vi "checkIfIsFromDirect.vi"(8 "error in (no error)":errorcluster, 10 "Game":refnum<class "Game.lvclass">, 11 "KickToBestRobotTactic in":refnum<class "KickToBestRobotTactic.lvclass">) -> (0 "error out":errorcluster, 2 "FromPreparePass":bool, 3 "KickToBestRobotTactic out":refnum<class "KickToBestRobotTactic.lvclass">)   [LabVIEW 2024, in "KickToBestRobotTactic.lvclass"]
uses:
  KickToBestRobotTactic.lvclass
  Game_class/Game.lvclass
  Game_class/Game.lvclass/Game.ctl
  Team_class/Team.lvclass/Team.ctl
  Playbook_class/Playbook.lvclass/Playbook.ctl
  5RobotsNormalGamePlay_class/5RobotsNormalGamePlay.lvclass/5RobotsNormalGamePlay.ctl
  5RobotsPassGamePlay_class/5RobotsPassGamePlay.lvclass/5RobotsPassGamePlay.ctl
  Playbook_class/Read offensive_plays.vi
  5RobotsNormalGamePlay_class/Read FromPreparePass.vi
  5RobotsPassGamePlay_class/Read FromPreparePass.vi
  Game_class/Read OffensiveTeam.vi
  Team_class/Read OffensivePlay.vi
  Ally_class/Ally.lvclass
  C:/Users/moise/Documents/GitHub/SSL_AI/Team_class/Team.lvclass
  Playbook_class/Playbook.lvclass
  Play_class/Play.lvclass
  TestPlay_class/TestPlay.lvclass
  EnemyPossessionAtEnemyFieldPlay_class/EnemyPossessionAtEnemyFieldPlay.lvclass
  EnemyPossessionAtOurFieldPlay_class/EnemyPossessionAtOurFieldPlay.lvclass
  NormalGamePlay_class/NormalGamePlay.lvclass
  IndirectEnemyPlay_class/IndirectEnemyPlay.lvclass
  PrepareKickoffAllyPlay_class/PrepareKickoffAllyPlay.lvclass
  PrepareKickoffEnemyPlay_class/PrepareKickoffEnemyPlay.lvclass
  KickPenaltyAllyPlay_class/KickPenaltyAllyPlay.lvclass
  PreparePenaltyAllyPlay_class/PreparePenaltyAllyPlay.lvclass
  DirectEnemyPlay_class/DirectEnemyPlay.lvclass
  PreparePenaltyEnemyPlay_class/PreparePenaltyEnemyPlay.lvclass
  BallOutOfFieldPlay_class/BallOutOfFieldPlay.lvclass
  StopOffensivePlay_class/StopOffensivePlay.lvclass
  PassPlay_class/PassPlay.lvclass
  DirectKickPlay_class/DirectKickPlay.lvclass
  HaltPlay_class/HaltPlay.lvclass
  PreparePassPlay_class/PreparePassPlay.lvclass
  PassToStriker_class/PassToStriker.lvclass
  PassTo2ndStriker_class/PassTo2ndStriker.lvclass
  SimplePass_class/SimplePass.lvclass
  PrepareRollToPassPlay_class/PrepareRollToPassPlay.lvclass
  PrepareDoublePassPlay_class/PrepareDoublePassPlay.lvclass
  TableWith2ndStrikerPlay_class/TableWith2ndStrikerPlay.lvclass
  TableWithStrikerPlay_class/TableWithStrikerPlay.lvclass
  PrepareTriplePassPlay_class/PrepareTriplePassPlay.lvclass
  ABCPassPlay_class/ABCPassPlay.lvclass
  PreparePassInGame1_class/PreparePassInGame1.lvclass
  ACBPassPlay_class/ACBPassPlay.lvclass
  PrepareKeeperPassPlay_class/PrepareKeeperPassPlay.lvclass
  KeeperPassToStrikerPlay_class/KeeperPassToStrikerPlay.lvclass
  5RobotsNormalGamePlay_class/5RobotsNormalGamePlay.lvclass
  5RobotsPassGamePlay_class/5RobotsPassGamePlay.lvclass
  5RobotsKeeperGame_class/5RobotsKeeperGame.lvclass
  5PreparePassGamePlay_class/5PreparePassGamePlay.lvclass
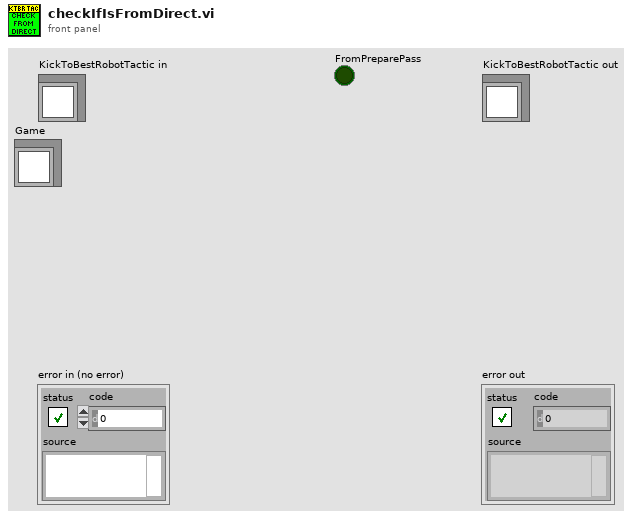
[diagram p1: front panel]
types:
  T1 = typedef "OffensivePlay.ctl" = enum16{"5RobotsPassGamePlay", "5PreparePassGame", "5RobotsKeeperGame", "KeeperPassToStriker", "5RobotsNormalGamePlay", "PrepareKeeperPass", "ACBPass", "ABCPass", "PrepareTriplePass", "TableWithStriker", "TableWith2ndStrikerPlay", "PrepareDoublePass", "PrepareRollToPass", "SimplePass", "PreparePass", "PassToStriker", "BallOutOfField", "PassTo2ndStriker", "StopOffensive", "Prepare Penalty Enemy", "EnemyPossessionAtEnemyField", "EnemyPossesionAtOurField", "TestPlay", "PreparePenaltyAlly", "KickPenaltyAlly", "PrepareKickoffAlly", "PrepareKickoffEnemy", "IndirectEnemy", "DirectEnemy", "PreparePassInGame1", "NormalGame", "DirectKick", "Pass", "Halt", "Timeout", "PassPlay", "PenaltyEnemy"}
  T2 = typedef "offensive_plays.ctl" = cluster{"Play":refnum<class "Play.lvclass">, "TestPlay":refnum<class "TestPlay.lvclass">, "EnemyPossessionAtEnemyFieldPlay":refnum<class "EnemyPossessionAtEnemyFieldPlay.lvclass">, "EnemyPossessionAtOurFieldPlay":refnum<class "EnemyPossessionAtOurFieldPlay.lvclass">, "NormalGamePlay":refnum<class "NormalGamePlay.lvclass">, "IndirectEnemyPlay":refnum<class "IndirectEnemyPlay.lvclass">, "PrepareKickoffAllyPlay":refnum<class "PrepareKickoffAllyPlay.lvclass">, "PrepareKickoffEnemyPlay":refnum<class "PrepareKickoffEnemyPlay.lvclass">, "KickPenaltyAllyPlay":refnum<class "KickPenaltyAllyPlay.lvclass">, "PreparePenaltyAllyPlay":refnum<class "PreparePenaltyAllyPlay.lvclass">, "DirectEnemyPlay":refnum<class "DirectEnemyPlay.lvclass">, "PreparePenaltyEnemyPlay":refnum<class "PreparePenaltyEnemyPlay.lvclass">, "BallOutOfFieldPlay":refnum<class "BallOutOfFieldPlay.lvclass">, "StopOffensivePlay":refnum<class "StopOffensivePlay.lvclass">, "PassPlay":refnum<class "PassPlay.lvclass">, "DirectKickPlay":refnum<class "DirectKickPlay.lvclass">, "HaltPlay":refnum<class "HaltPlay.lvclass">, "PreparePassPlay":refnum<class "PreparePassPlay.lvclass">, "PassToStrikerPlay":refnum<class "PassToStriker.lvclass">, "PassTo2ndStrikerPlay":refnum<class "PassTo2ndStriker.lvclass">, "SimplePassPlay":refnum<class "SimplePass.lvclass">, "PrepareRollToPassPlay":refnum<class "PrepareRollToPassPlay.lvclass">, "PrepareDoublePassPlay":refnum<class "PrepareDoublePassPlay.lvclass">, "TableWith2ndStrikerPlay":refnum<class "TableWith2ndStrikerPlay.lvclass">, "TableWithStrikerPlay":refnum<class "TableWithStrikerPlay.lvclass">, "PrepareTriplePassPlay":refnum<class "PrepareTriplePassPlay.lvclass">, "ABCPassPlay":refnum<class "ABCPassPlay.lvclass">, "PreparePassInGame1":refnum<class "PreparePassInGame1.lvclass">, "ACBPassPlay":refnum<class "ACBPassPlay.lvclass">, "PrepareKeeperPassPlay":refnum<class "PrepareKeeperPassPlay.lvclass">, "KeeperPassToStrikerPlay":refnum<class "KeeperPassToStrikerPlay.lvclass">, "SimplePass":refnum<class "SimplePass.lvclass">, "SimplePass 2":refnum<class "SimplePass.lvclass">, "5RobotsNormalGamePlay":refnum<class "5RobotsNormalGamePlay.lvclass">, "5RobotsPassGamePlay":refnum<class "5RobotsPassGamePlay.lvclass">, "5RobotsKeeperGame":refnum<class "5RobotsKeeperGame.lvclass">, "5PreparePassGamePlay":refnum<class "5PreparePassGamePlay.lvclass">}
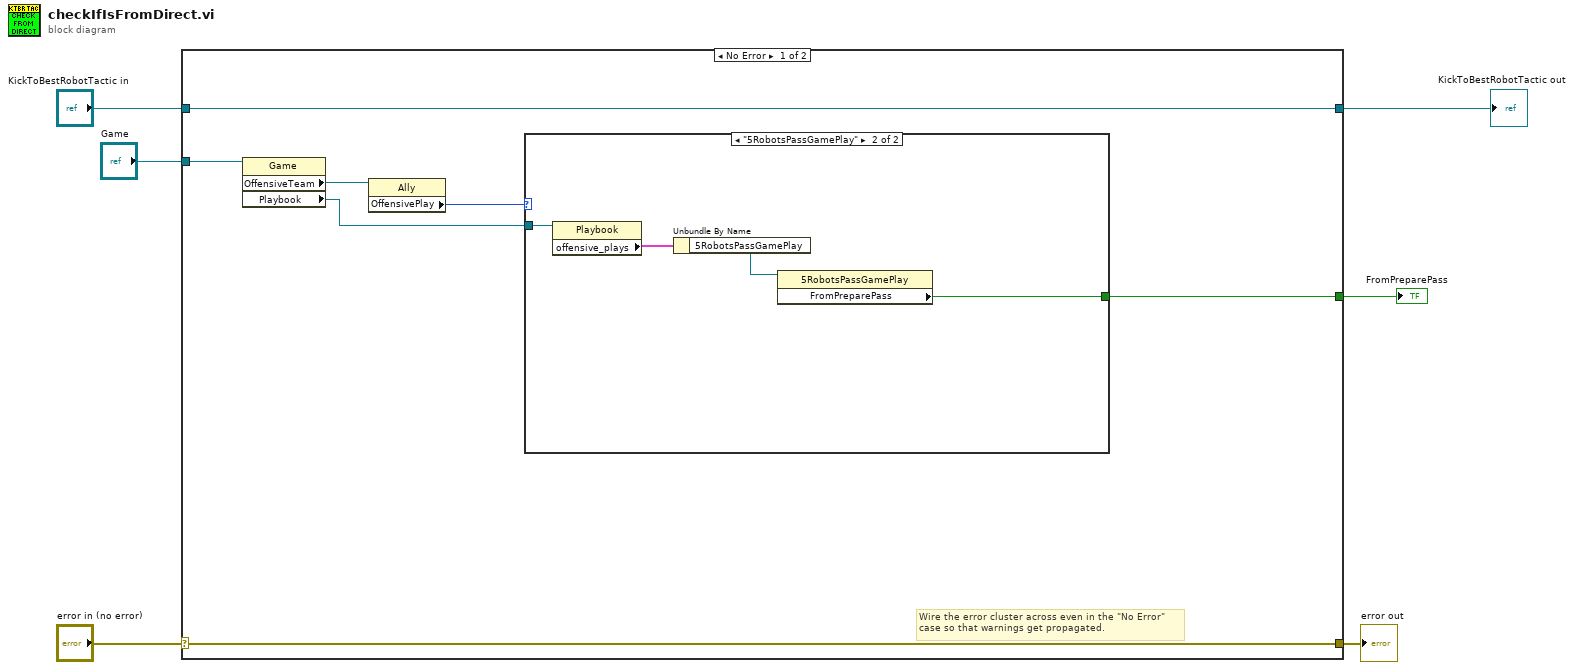
[diagram p0: block diagram]
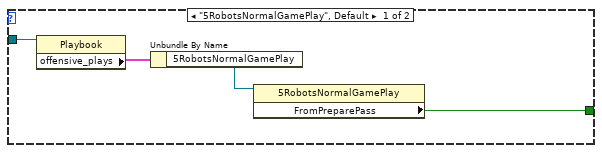
[diagram p2: hidden frame]
diagram:
  n1 = case shown="No Error" "error in (no error)" {
    selector: "error in (no error)" -> [w12 w23]
    tunnel: [w12 w23] -> w5
    tunnel: [w13 w22] -> w3
    tunnel: "KickToBestRobotTactic in" -> [w13 w22]
    tunnel: "Game" -> [w11 _]
    tunnel: [w7 _] -> w1
    frame No Error {
      # "Wire the error cluster across even in the \"No Error\"\ncase so that warnings get propagated."
      n2 = property class="Game"(reference=w11) -> ("OffensiveTeam"=w10:refnum<class "Ally.lvclass">, "Playbook"=w8:refnum<class "Playbook.lvclass">)  [unwired: 1 in, 2 out]
      n3 = property class="Ally"(reference=w10) -> ("OffensivePlay"=w9:T1)  [unwired: 1 in, 2 out]
      n4 = case shown="\"5RobotsPassGamePlay\"" w9 {
        tunnel: w8 -> [w17 w21]
        tunnel: [w14 w18] -> w7
        frame "5RobotsNormalGamePlay", Default {
          n5 = property class="Playbook"(reference=w17) -> ("offensive_plays"=w16:T2)  [unwired: 1 in, 2 out]
          n6 = Unbundle By Name(w16) -> ("5RobotsNormalGamePlay"=w15:refnum<class "5RobotsNormalGamePlay.lvclass">)
          n7 = property class="5RobotsNormalGamePlay"(reference=w15) -> ("FromPreparePass"=w14:bool)  [unwired: 1 in, 2 out]
        }
        frame "5RobotsPassGamePlay" {
          n8 = property class="Playbook"(reference=w21) -> ("offensive_plays"=w20:T2)  [unwired: 1 in, 2 out]
          n9 = Unbundle By Name(w20) -> ("5RobotsPassGamePlay"=w19:refnum<class "5RobotsPassGamePlay.lvclass">)
          n10 = property class="5RobotsPassGamePlay"(reference=w19) -> ("FromPreparePass"=w18:bool)  [unwired: 1 in, 2 out]
        }
      }
    }
    frame Error {
    }
  }
  "error out" <- w5
  "KickToBestRobotTactic out" <- w3
  "FromPreparePass" <- w1
